vi "Remove zeros from the end of fractional string number.vi"(1 "Strings Array":string[](array[string])) -> (0 "Filtered Strings Array":string[](array[string]))   [LabVIEW 2020]
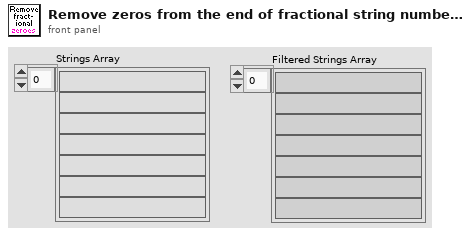
[diagram p1: front panel]
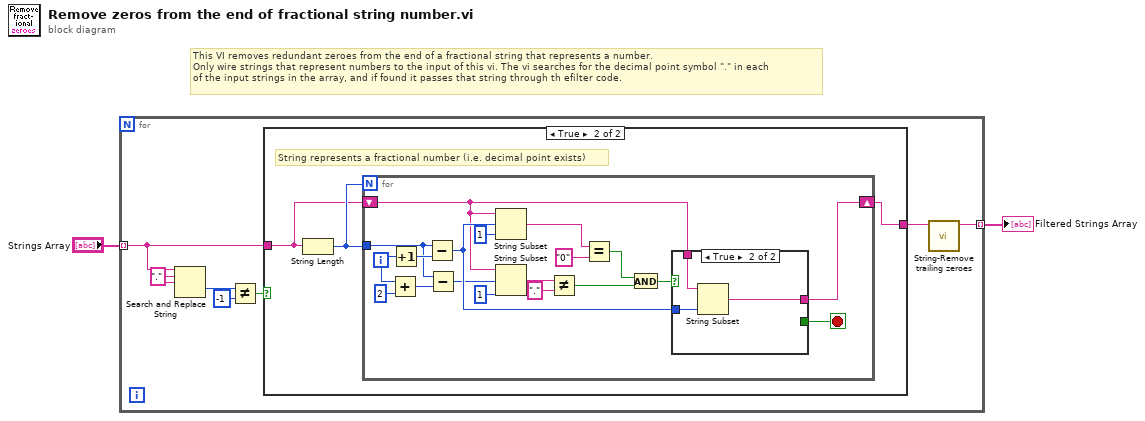
[diagram p0: block diagram]
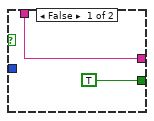
[diagram p3: hidden frame]
diagram:
  # "This VI removes redundant zeroes from the end of a fractional string that represents a number.\nOnly wire strings that represent numbers to the input of this vi. The vi searches for the decimal point symbol \".\" in each \nof the input strings in the array, and if found it passes that string through th efilter code."
  n1 = for {
    tunnel: "Strings Array" -> [w9] mode=indexing
    tunnel: [w3] -> w1 mode=indexing
    w8 = "." ("search string")
    n2 = Search and Replace String(input string=w9, search string=w8, replace string=w8) -> (offset past replacement=w7:i32)  [unwired: 5 in, 3 out]
    n3 = Not Equal?(x=w7, y=-1) -> (x != y?=w5:bool)
    n4 = case shown="True" w5 {
      tunnel: w9 -> [w10 w11]
      tunnel: [w10 w12] -> w4
      frame False {
      }
      frame True {
        # "String represents a fractional number (i.e. decimal point exists)"
        n5 = String Length(string=w11) -> (length=w13:i32)
        n6 = for {
          N: w13 -> [_]
          tunnel: w13 -> [w16]
          shift-right: [w18] -> w12
          shift-left: w11 -> [w17]
          i -> [w29]
          stop <- w19 stop-if-true
          n7 = Add(x=w29, y=2) -> (x+y=w15:i32)
          n8 = Increment(x=w29) -> (x+1=w31:i32)
          n9 = Subtract(x=w16, y=w31) -> (x-y=w23:i32)
          n10 = Subtract(x=w16, y=w15) -> (x-y=w14:i32)
          n11 = String Subset(string=w17, offset (0)=w23, length (rest)=1 ("length (rest)")) -> (substring=w25:string)
          n12 = String Subset(string=w17, offset (0)=w14, length (rest)=1 ("length (rest)")) -> (substring=w27:string)
          n13 = Not Equal?(x=w27, y=".") -> (x != y?=w21:bool)
          n14 = Equal?(x=w25, y="0") -> (x = y?=w22:bool)
          n15 = And(x=w22, y=w21) -> (x .and. y?=w20:bool)
          n16 = case shown="True" w20 {
            tunnel: w23 -> [_ w37]
            tunnel: [w33 w36] -> w18
            tunnel: w17 -> [w33 w35]
            tunnel: [TRUE _] -> w19
            frame False {
            }
            frame True {
              n17 = String Subset(string=w35, length (rest)=w37) -> (substring=w36:string)  [unwired: 1 in]
            }
          }
        }
      }
    }
    n18 = call "String-Remove trailing zeroes.vi"("String in"=w4) -> ("String out"=w3:string)  [unwired: 10 in]
  }
  "Filtered Strings Array" <- w1
